vi "Imagen.vi"   [LabVIEW 2016]
uses:
  <vilib>/picture/3D Picture Control/Object/Create Object (name).vi
  <vilib>/picture/3D Picture Control/Object/Add Object (no reference).vi
  <vilib>/picture/3D Picture Control/NI_3D Picture Control.lvlib
types:
  T1 = enum16{"Points", "Lines", "Line Strip", "Line Loop", "Triangles", "Triangle Strip", "Triangle Fan", "Quads", "Quad Strip", "Polygon"}
  T2 = enum16{"Overall", "Per Primitive", "Per Vertex", "Binding Off"}
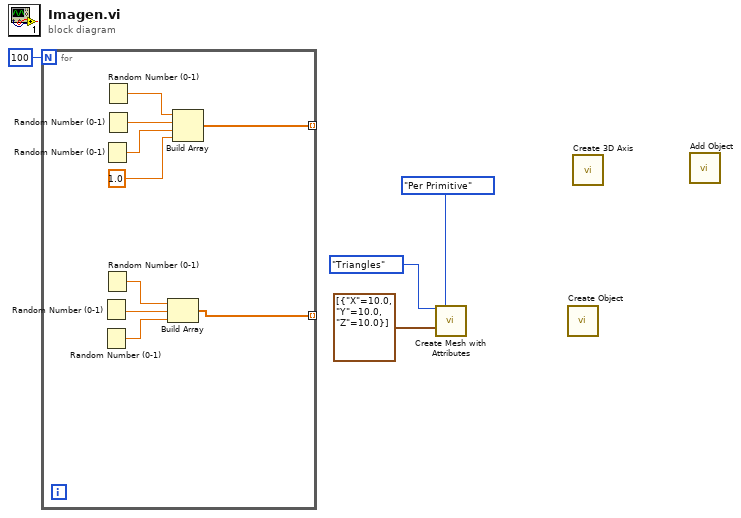
[diagram p0: block diagram]
diagram:
  n1 = for {
    N: 100 -> [_]
    tunnel: [w6] -> _ mode=indexing
    tunnel: [w5] -> _ mode=indexing
    n2 = Random Number (0-1)() -> (number: 0 to 1=w9:dbl)
    n3 = Random Number (0-1)() -> (number: 0 to 1=w7:dbl)
    n4 = Random Number (0-1)() -> (number: 0 to 1=w13:dbl)
    n5 = Random Number (0-1)() -> (number: 0 to 1=w8:dbl)
    n6 = Random Number (0-1)() -> (number: 0 to 1=w11:dbl)
    n7 = Random Number (0-1)() -> (number: 0 to 1=w12:dbl)
    n8 = Build Array(w8, w9, w7) -> (w5:dbl[])
    n9 = Build Array(w11, w12, w13, 1.0 ("element")) -> (w6:dbl[])
  }
  n10 = call <vilib>:"Create Mesh with Attributes.vi"("Draw Mode"=T1."Triangles", "Color Binding Mode"=T2."Per Primitive", "Normal Array"=cluster{"X":sgl, "Y":sgl, "Z":sgl}[] [{"X"=10.0, "Y"=10.0, "Z"=10.0}]) -> ()  [unwired: 11 in, 2 out]
  n11 = call-poly <vilib>:"Create Object.vi"() -> ()  [unwired: 10 in, 2 out]
  n12 = call <vilib>:"Create 3D Axis.vi"() -> ()  [unwired: 10 in, 2 out]
  n13 = call-poly <vilib>:"Add Object.vi"() -> ()  [unwired: 10 in, 2 out]
